vi "Flow Control Wait.vi"(2 "milliseconds to wait":u32, 3 "error in (no error)":errorcluster) -> (17 "error out":errorcluster)   [LabVIEW 2014]
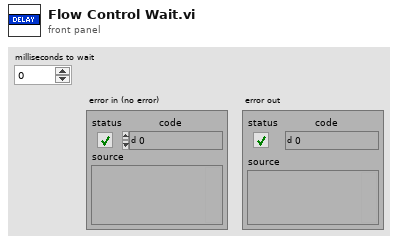
[diagram p1: front panel]
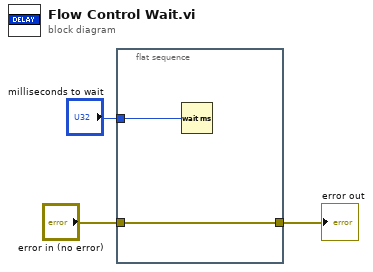
[diagram p0: block diagram]
diagram:
  n1 = flat-sequence {
    tunnel: "milliseconds to wait" -> [w5]
    tunnel: [w4] -> w2
    tunnel: "error in (no error)" -> [w4]
    frame #0 {
      n2 = Wait (ms)(milliseconds to wait=w5) -> ()  [unwired: 1 out]
    }
  }
  "error out" <- w2
